vi "estrutura_case.vi"() -> ()   [LabVIEW 2020]
panel:
  in  "String":string
  in  "Operacao":i8
  in  "stop":bool
  out "resultado":dbl
  in  "Dado B":dbl
  in  "Dado A":dbl
  # "0 - A -B\n1 - A+B\n2 - AxB"
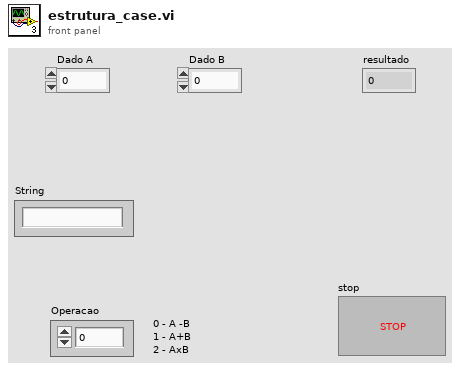
[diagram p1: front panel]
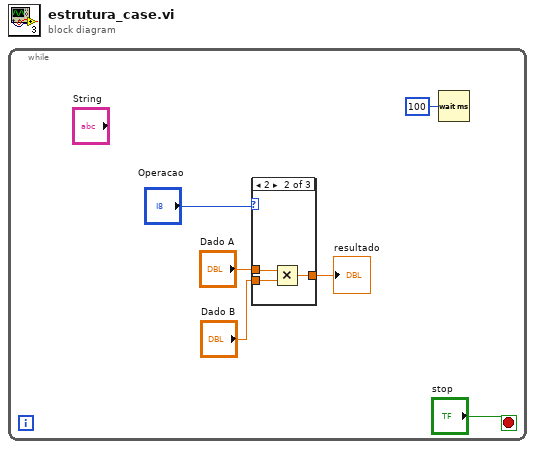
[diagram p0: block diagram]
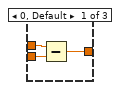
[diagram p2: hidden frame]
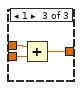
[diagram p3: hidden frame]
diagram:
  n1 = while {
    stop <- "stop" stop-if-true
    n2 = case shown="2" "Operacao" {
      tunnel: "Dado A" -> [w9 w10 w14]
      tunnel: "Dado B" -> [w8 w11 w15]
      tunnel: [w7 w12 w13] -> w4
      frame 0, Default {
        n3 = Subtract(x=w9, y=w8) -> (x-y=w7:dbl)
      }
      frame 2 {
        n4 = Multiply(x=w10, y=w11) -> (x*y=w12:dbl)
      }
      frame 1 {
        n5 = Add(x=w14, y=w15) -> (x+y=w13:dbl)
      }
    }
    "resultado" <- w4
    n6 = Wait (ms)(milliseconds to wait=u32 100) -> ()  [unwired: 1 out]
  }
